vi "Show Project Window.vi"(6 "Variant in":variant, 7 "Shift Pressed?":bool, 8 "error in (no error)":errorcluster, 10 "QD Combo Box Ref":refnum<vi>, 11 "QD Launch VI Ref":refnum<vi>) -> (0 "error out":errorcluster, 4 "Variant out":variant)   [LabVIEW 2013]
doc: "This shortcut shows active project window.\n\nDefault Shortcut - [j]"
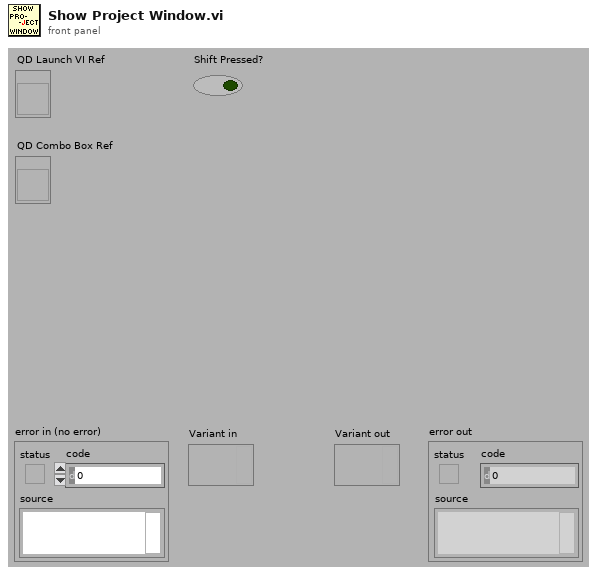
[diagram p1: front panel]
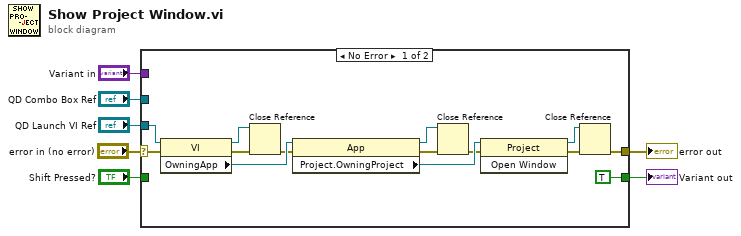
[diagram p0: block diagram]
diagram:
  n1 = case shown="No Error" "error in (no error)" {
    selector: "error in (no error)" -> [w19 w22]
    tunnel: [w8 w22] -> w6
    tunnel: "QD Launch VI Ref" -> [w18 _]
    tunnel: "Shift Pressed?" -> [_ _]
    tunnel: "QD Combo Box Ref" -> [_ _]
    tunnel: "Variant in" -> [_ _]
    tunnel: [TRUE _] -> w1
    frame No Error {
      n2 = property class="VI"(reference=w18, error in=w19) -> (reference out=w16:refnum<vi>, error out=w17:errorcluster, "OwningApp"=w15:refnum<vi>)
      n3 = Close Reference(reference=w16, error in (no error)=w17) -> (error out=w14:errorcluster)
      n4 = property class="App"(reference=w15, error in=w14) -> (reference out=w12:refnum<vi>, error out=w13:errorcluster, "Project.OwningProject"=w20:refnum<vi>)
      n5 = Close Reference(reference=w12, error in (no error)=w13) -> (error out=w11:errorcluster)
      n6 = invoke class="Project" method="Open Window"(reference=w20, error in=w11) -> (reference out=w9:refnum<vi>, error out=w10:errorcluster)  [unwired: 1 in, 1 out]
      n7 = Close Reference(reference=w9, error in (no error)=w10) -> (error out=w8:errorcluster)
    }
    frame Error {
    }
  }
  "error out" <- w6
  "Variant out" <- w1
